vi "Configure and Source Pin.vi"(0 "NI Digital in":refnum<k15>, 5 "Source Pin Configuration":T1={"Pin Name"="", "Pin Output Function"=1300, "Voltage (V)"=1.8, "Current (A)"=0.2} {"Pin Output Function" items=["DC Voltage"=1300, "DC Current"=1301]}, 11 "error in (no error)":errorcluster) -> (4 "NI Digital out":refnum<k15>, 15 "error out":errorcluster)   [LabVIEW 2016, in "Digital.lvlib"]
uses:
  Digital.lvlib
  <instrlib>/niDigital/niDigital.llb/niDigital Output Function.ctl
  Type Definitions/Source Pin Configuration.ctl
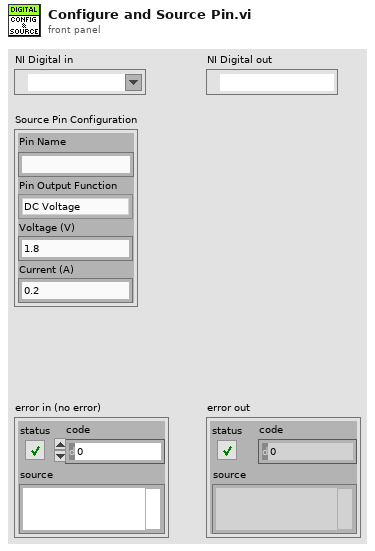
[diagram p1: front panel]
types:
  T1 = typedef "Digital.lvlib/Source Pin Configuration.ctl" = cluster{"Pin Name":string, "Pin Output Function":T2, "Voltage (V)":dbl, "Current (A)":dbl}
  T2 = typedef "niDigital Output Function.ctl" = i32
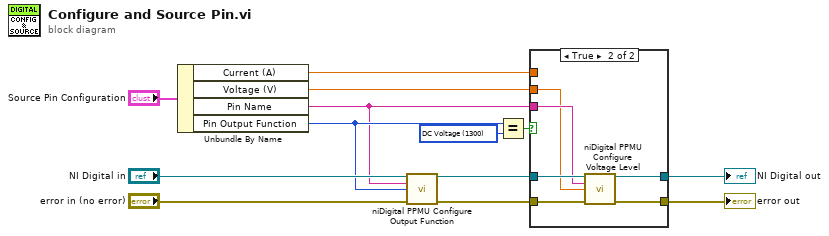
[diagram p0: block diagram]
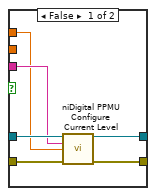
[diagram p2: hidden frame]
diagram:
  w3 = T2 1300 items=["DC Voltage"=1300, "DC Current"=1301] ("Pin Output Function")
  n1 = Unbundle By Name("Source Pin Configuration") -> ("Current (A)"=w5:dbl, "Voltage (V)"=w6:dbl, "Pin Name"=w1:string, "Pin Output Function"=w4:T2)
  n2 = call <instrlib>:"niDigital PPMU Configure Output Function.vi"("instrument handle"="NI Digital in", "channel list"=w1, "output function"=w4, "error in"="error in (no error)") -> ("instrument handle out"=w8:refnum<k15>, "error out"=w11:errorcluster)  [unwired: 10 in]
  n3 = Equal?(x=w4, y=w3) -> (x = y?=w2:bool)
  n4 = case shown="True" w2 {
    tunnel: w11 -> [w19 w25]
    tunnel: [w18 w24] -> w9
    tunnel: w8 -> [w17 w23]
    tunnel: [w16 w22] -> w7
    tunnel: w6 -> [_ w20]
    tunnel: w5 -> [w14 _]
    tunnel: w1 -> [w15 w21]
    frame False {
      n5 = call <instrlib>:"niDigital PPMU Configure Current Level.vi"("instrument handle"=w17, "channel list"=w15, "current level (A)"=w14, "error in"=w19) -> ("instrument handle out"=w16:refnum<k15>, "error out"=w18:errorcluster)  [unwired: 10 in]
    }
    frame True {
      n6 = call <instrlib>:"niDigital PPMU Configure Voltage Level.vi"("instrument handle"=w23, "channel list"=w21, "voltage level (V)"=w20, "error in"=w25) -> ("instrument handle out"=w22:refnum<k15>, "error out"=w24:errorcluster)  [unwired: 10 in]
    }
  }
  "NI Digital out" <- w7
  "error out" <- w9
